vi "ToCowlAngle.vi"(1 "Initial Angle(Degrees)":dbl, 2 "Input(Encoder Units)":dbl) -> (0 "Angle(Degrees)":dbl)   [LabVIEW 2019]
panel:
  in  "conversion factor":dbl
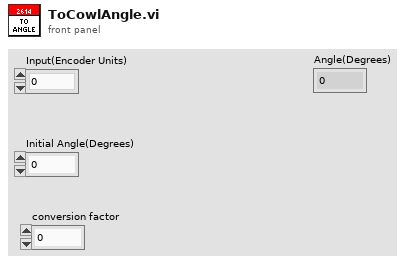
[diagram p1: front panel]
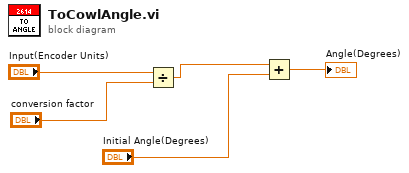
[diagram p0: block diagram]
diagram:
  n1 = Divide(x="Input(Encoder Units)", y="conversion factor") -> (x/y=w2:dbl)
  n2 = Add(x=w2, y="Initial Angle(Degrees)") -> (x+y=→"Angle(Degrees)":dbl)
